vi "splid2imagesFromArray.vi"(8 "Beam in":T1, 10 "Combined array":u8[][][](array[numeric]), 11 "Image in":T1) -> (0 "Beam Out":T1, 3 "Image out":T1)   [LabVIEW 2022 SP3]
uses:
  <vilib>/vision/Image Controls.llb/IMAQ Image.ctl
  <vilib>/vision/NI_Vision_Development_Module.lvlib
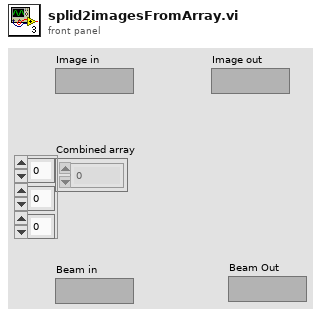
[diagram p1: front panel]
types:
  T1 = typedef "IMAQ Image.ctl" = refnum<image>
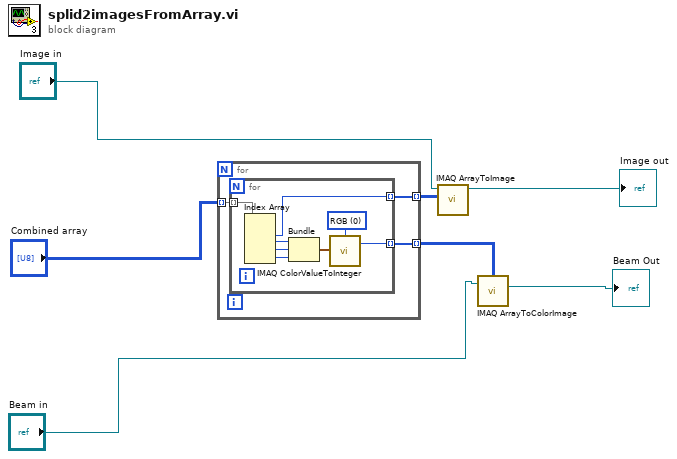
[diagram p0: block diagram]
diagram:
  n1 = for {
    tunnel: "Combined array" -> [w10] mode=indexing
    tunnel: [w9] -> w6 mode=indexing
    tunnel: [w8] -> w1 mode=indexing
    n2 = for {
      tunnel: w10 -> [w18] mode=indexing
      tunnel: [w17] -> w9 mode=indexing
      tunnel: [w16] -> w8 mode=indexing
      w15 = u16 0 items=["RGB", "HSL", "HSV", "HSI"] ("Color Mode")
      n3 = Index Array(array=w18) -> (element #1=w17:u8, element #2=w13:u8, element #3=w12:u8, element #4=w11:u8)  [unwired: 4 in]
      n4 = Bundle(w13, w12, w11) -> (w14:cluster{u8, u8, u8})  [unwired: 1 in]
      n5 = call "IMAQ ColorValueToInteger"("Color Value"=w14, "Color Mode"=w15) -> ("U32 value"=w16:u32)  [unwired: 3 in, 3 out]
    }
  }
  n6 = call "IMAQ ArrayToImage"("Image Pixels (U8)"=w6, "Image"="Image in") -> ("Image Out"=→"Image out":T1)  [unwired: 8 in, 1 out]
  n7 = call "IMAQ ArrayToColorImage"("Image Pixels (U32)"=w1, "Image"="Beam in") -> ("Image Out"=→"Beam Out":T1)  [unwired: 3 in, 1 out]
